vi "Refresh FPGA Bitfile.vi"(8 "error in (no error)":errorcluster, 11 "Node Ptr":u64 format="%.0x") -> (0 "error out":errorcluster)   [LabVIEW 2013, in "Engine Simulation Toolkit System Explorer.lvlib"]
uses:
  Engine Simulation Toolkit System Explorer.lvlib
  Shared/Properties.vi
  <vilib>/NI Veristand/Custom Device API/Get Item Property (Dependent File).vi
  Shared/Constants and GUIDs.vi
  <vilib>/NI Veristand/Custom Device API/Set Item Property (Dependent File).vi
  Shared/Engine Simulation Toolkit Shared.lvlib
  <vilib>/NI Veristand/Custom Device API/Custom Device API.lvlib
panel:
  in  "Tag":string
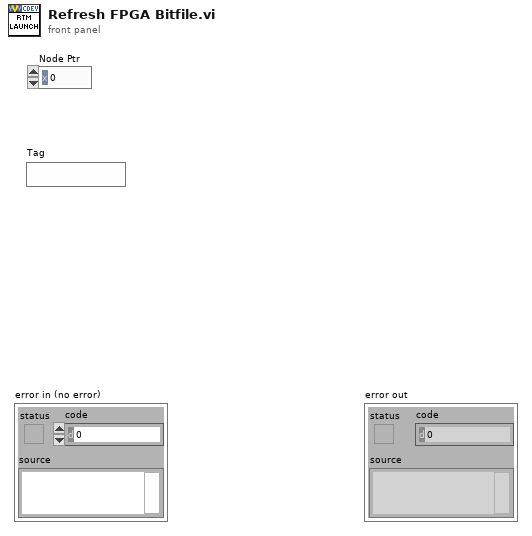
[diagram p1: front panel]
types:
  T1 = typedef "Custom Device API.lvlib/Custom Device Item Ref.ctl" = u64
  T2 = typedef "Custom Device API.lvlib/Dependent File Optional Info.ctl" = cluster{"Version":string, "RTDestination":path, "ForceDownload":bool, "SupportedTarget":string, "MD5":string}
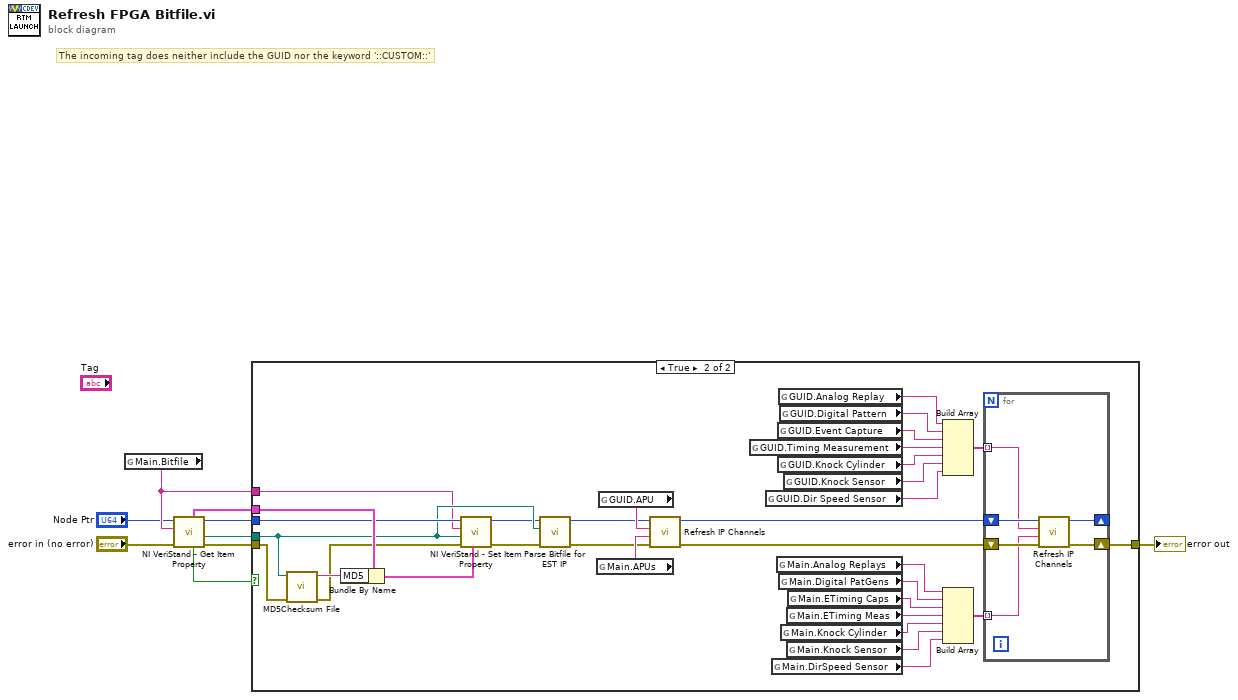
[diagram p0: block diagram]
diagram:
  # "The incoming tag does neither include the GUID nor the keyword '::CUSTOM::'"
  n1 = global read "Properties.vi" "Main.Bitfile"() -> (w4:string)
  n2 = call-poly <vilib>:"NI VeriStand - Get Item Property.vi"("error in (no error)"="error in (no error)", "Property Name"=w4, "Item Ref in"="Node Ptr") -> ("error out"=w7:errorcluster, "Path"=w8:path, "Item Ref out"=w5:T1, "Found"=w9:bool, "OptionalInfo"=w6:T2)  [unwired: 4 in]
  n3 = case shown="True" w9 {
    tunnel: w8 -> [_ w37]
    tunnel: w7 -> [w10 w39]
    tunnel: w6 -> [_ w42]
    tunnel: w5 -> [_ w38]
    tunnel: [w10 w18] -> w1
    tunnel: w4 -> [_ w11]
    frame False {
    }
    frame True {
      n4 = call <vilib>:"MD5Checksum File.vi"("error in (no error)"=w39, "Path"=w37) -> ("error out"=w40:errorcluster, "MD5 message-digest"=w43:string)  [unwired: 8 in]
      n5 = Bundle By Name(cluster=w42, "MD5"=w43) -> (w41:T2)
      n6 = call-poly <vilib>:"NI VeriStand - Set Item Property.vi"("OptionalInfo"=w41, "error in (no error)"=w40, "Path"=w37, "Property Name"=w11, "Item Ref in"=w38) -> ("error out"=w36:errorcluster, "Item Ref out"=w35:T1)  [unwired: 4 in, 1 out]
      n7 = call "Parse Bitfile for EST IP.vi"("error in (no error)"=w36, "bitfile path"=w37, "Item Ref in"=w35) -> ("error out"=w15:errorcluster, "Item Ref out"=w14:T1)  [unwired: 5 in, 2 out]
      n8 = global read "Properties.vi" "Main.APUs"() -> (w16:string)
      n9 = global read "Constants and GUIDs.vi" "GUID.APU"() -> (w17:string)
      n10 = call "Refresh IP Channels.vi"("error in (no error)"=w15, "Main"=w16, "GUID"=w17, "Section Ref in"=w14) -> ("error out"=w13:errorcluster, "Section Ref out"=w12:T1)  [unwired: 6 in]
      n11 = global read "Constants and GUIDs.vi" "GUID.Timing Measurement"() -> (w30:string)
      n12 = global read "Constants and GUIDs.vi" "GUID.Dir Speed Sensor"() -> (w29:string)
      n13 = global read "Properties.vi" "Main.DirSpeed Sensor"() -> (w22:string)
      n14 = global read "Properties.vi" "Main.Analog Replays"() -> (w28:string)
      n15 = global read "Constants and GUIDs.vi" "GUID.Event Capture"() -> (w31:string)
      n16 = global read "Constants and GUIDs.vi" "GUID.Knock Cylinder"() -> (w20:string)
      n17 = global read "Constants and GUIDs.vi" "GUID.Analog Replay"() -> (w33:string)
      n18 = global read "Properties.vi" "Main.Digital PatGens"() -> (w27:string)
      n19 = global read "Constants and GUIDs.vi" "GUID.Digital Pattern"() -> (w32:string)
      n20 = global read "Properties.vi" "Main.Knock Cylinder"() -> (w24:string)
      n21 = global read "Constants and GUIDs.vi" "GUID.Knock Sensor"() -> (w19:string)
      n22 = global read "Properties.vi" "Main.ETiming Meas"() -> (w25:string)
      n23 = global read "Properties.vi" "Main.Knock Sensor"() -> (w23:string)
      n24 = global read "Properties.vi" "Main.ETiming Caps"() -> (w26:string)
      n25 = Build Array(w33, w32, w31, w30, w20, w19, w29) -> (w34:string[])
      n26 = Build Array(w28, w27, w26, w25, w24, w23, w22) -> (w21:string[])
      n27 = for {
        tunnel: w34 -> [w45] mode=indexing
        shift-right: [w47] -> w18
        shift-left: w13 -> [w49]
        shift-right: [w48] -> _
        shift-left: w12 -> [w46]
        tunnel: w21 -> [w44] mode=indexing
        n28 = call "Refresh IP Channels.vi"("error in (no error)"=w49, "Main"=w44, "GUID"=w45, "Section Ref in"=w46) -> ("error out"=w47:errorcluster, "Section Ref out"=w48:T1)  [unwired: 6 in]
      }
    }
  }
  "error out" <- w1
